vi "Blink_SDK_example.vi"() -> ()   [LabVIEW 2010]
uses:
  Blink_C_wrapper.dll
  ImageGen.dll
panel:
  out "ImgData 2":u8[](array[numeric])
  in  "Wait Timer":dbl=1000.0
  in  "Use External Triggers":bool
  out "BoardNum":i32
  out "ImgData":u8[](array[numeric])
  # "PCIe  LabVIEWSDK"
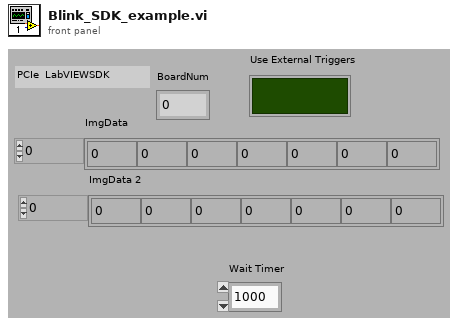
[diagram p1: front panel]
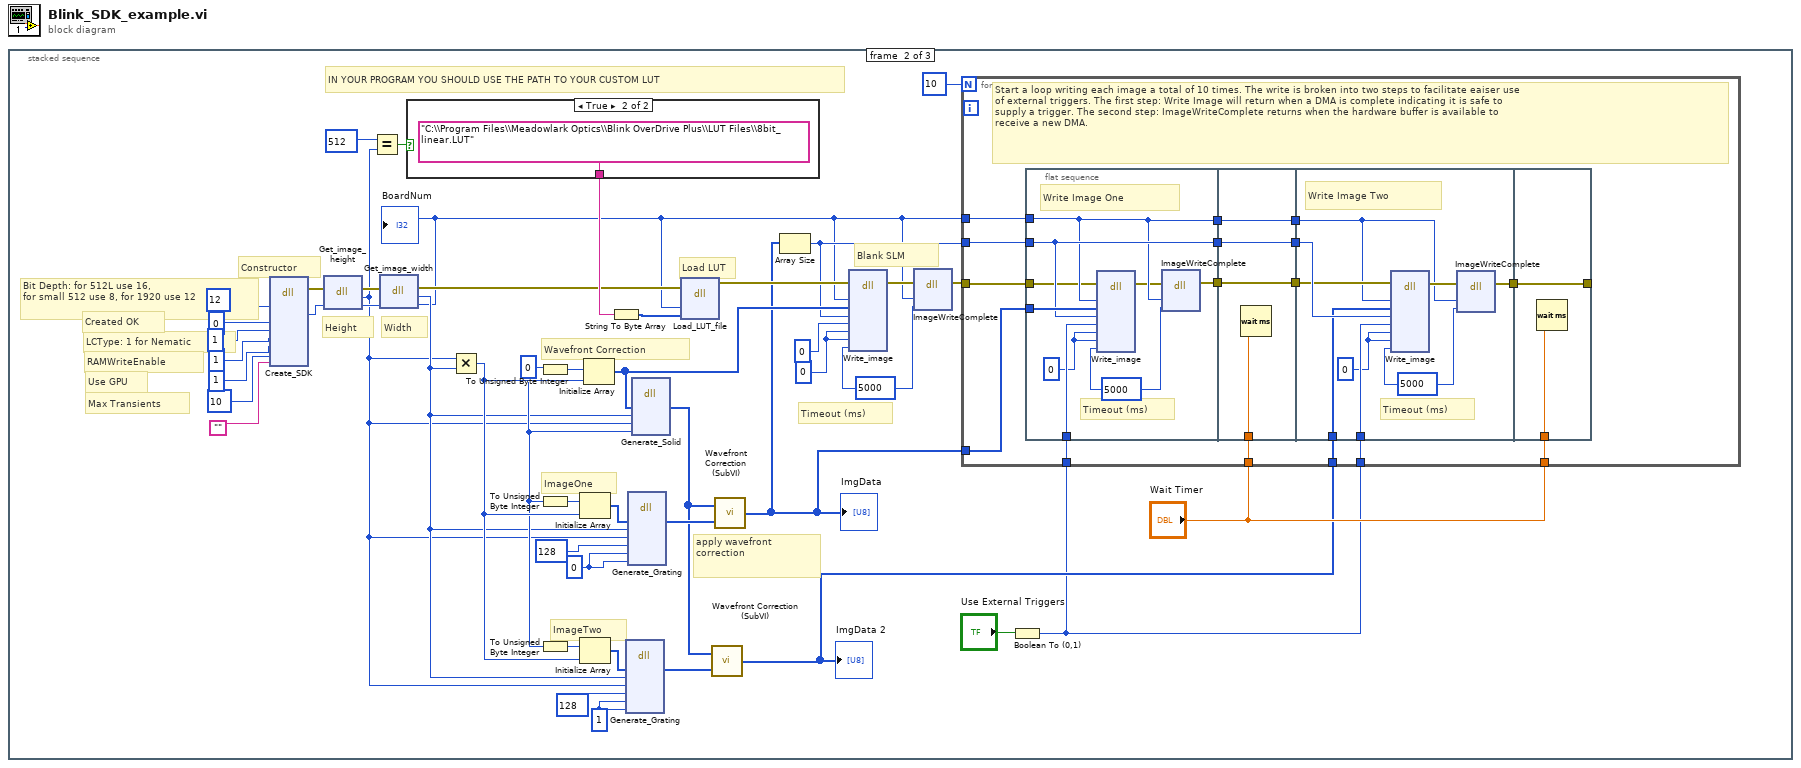
[diagram p0: block diagram]
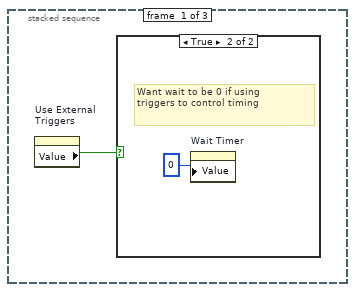
[diagram p2: hidden frame]
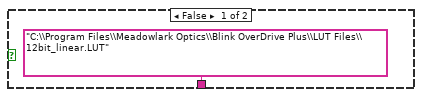
[diagram p4: hidden frame]
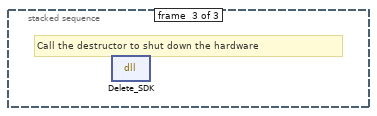
[diagram p5: hidden frame]
diagram:
  n1 = stacked-sequence {
    frame #0 {
      n2 = property on="Use External \nTriggers" class="Bool (strict)"() -> ("Value"=w1:bool)  [unwired: 2 in, 2 out]
      n3 = case shown="True" w1 {
        frame False {
        }
        frame True {
          # "Want wait to be 0 if using \ntriggers to control timing"
          n4 = property on="Wait Timer" class="DigNum (strict)"("Value"=0) -> ()  [unwired: 2 in, 2 out]
        }
      }
    }
    frame #1 {
      w14 = 5000
      w3 = 0
      w29 = 1
      w31 = 0
      w34 = 0
      # "Timeout (ms)"
      # "Blank SLM"
      # "IN YOUR PROGRAM YOU SHOULD USE THE PATH TO YOUR CUSTOM LUT"
      # "Load LUT"
      # "ImageTwo"
      # "ImageOne"
      # "Wavefront Correction"
      # "Width"
      # "Height"
      # "apply wavefront\ncorrection"
      # "Created OK"
      # "Max Transients"
      # "Use GPU"
      # "RAMWriteEnable"
      # "Bit Depth: for 512L use 16, \nfor small 512 use 8, for 1920 use 12"
      # "LCType: 1 for Nematic"
      # "Constructor"
      n5 = dll-call lib="C:/Meadowlark/Repos-git/MeadowlarkOverdrivePlus/src/Blink_SDK_example_grizzly/Blink_C_wrapper.dll" fn="Create_SDK"("SLM_bit_depth"=12, "constructed_ok"=0, "is_nematic_type"=1, "RAM_write_enable"=1, "use_GPU_if_available"=1, "max_transient_frames"=10, "static_regional_lut_file"="") -> (error out=w17:errorcluster, "n_boards_found"=w16:u64)  [unwired: 12 in, 1 out]
      n6 = dll-call lib="C:/Meadowlark/Repos-git/MeadowlarkOverdrivePlus/src/Blink_SDK_example_grizzly/Blink_C_wrapper.dll" fn="Get_image_height"(error in=w17, "Board"=w16) -> (error out=w39:errorcluster, "return type"=w20:i32, "Board"=w40:u32)  [unwired: 2 in, 1 out]
      n7 = Equal?(x=512, y=w20) -> (x = y?=w22:bool)
      n8 = dll-call lib="C:/Meadowlark/Repos-git/MeadowlarkOverdrivePlus/src/Blink_SDK_example_grizzly/Blink_C_wrapper.dll" fn="Get_image_width"(error in=w39, "Board"=w40) -> (error out=w12:errorcluster, "return type"=w27:i32, "Board"=w4:u32)  [unwired: 2 in, 1 out]
      "BoardNum" <- w4
      n9 = case shown="True" w22 {
        tunnel: ["C:\\Program Files\\Meadowlark Optics\\Blink OverDrive Plus\\LUT Files\\12bit_linear.LUT" "C:\\Program Files\\Meadowlark Optics\\Blink OverDrive Plus\\LUT Files\\8bit_linear.LUT"] -> w19
        frame False {
        }
        frame True {
        }
      }
      n10 = Multiply(x=w20, y=w27) -> (x*y=w38:i32)
      n11 = To Unsigned Byte Integer(number=w34) -> (unsigned 8bit integer=w37:u8)
      n12 = To Unsigned Byte Integer(number=w34) -> (unsigned 8bit integer=w36:u8)
      n13 = To Unsigned Byte Integer(number=w34) -> (unsigned 8bit integer=w35:u8)
      n14 = Initialize Array(w36, w38) -> (w33:u8[])
      n15 = Initialize Array(w35, w38) -> (w30:u8[])
      n16 = Initialize Array(w37, w38) -> (w9:u8[])
      n17 = String To Byte Array(string=w19) -> (unsigned byte array=w18:u8[])
      n18 = dll-call lib="C:/Meadowlark/Repos-git/MeadowlarkOverdrivePlus/src/Blink_SDK_example_grizzly/ImageGen.dll" fn="Generate_Grating"("Array"=w30, "Width"=w27, "Height"=w20, "Period"=128, "Increasing"=w29, "Horizontal"=w29) -> ("Array"=w24:u8[])  [unwired: 9 in, 2 out]
      n19 = dll-call lib="C:/Meadowlark/Repos-git/MeadowlarkOverdrivePlus/src/Blink_SDK_example_grizzly/ImageGen.dll" fn="Generate_Grating"("Array"=w33, "Width"=w27, "Height"=w20, "Period"=128, "Increasing"=w31, "Horizontal"=w31) -> ("Array"=w26:u8[])  [unwired: 9 in, 2 out]
      n20 = dll-call lib="C:/Meadowlark/Repos-git/MeadowlarkOverdrivePlus/src/Blink_SDK_example_grizzly/ImageGen.dll" fn="Generate_Solid"("Array"=w9, "Width"=w27, "Height"=w20, "PixelValue"=w34) -> ("Array"=w25:u8[])  [unwired: 7 in, 2 out]
      n21 = dll-call lib="C:/Meadowlark/Repos-git/MeadowlarkOverdrivePlus/src/Blink_SDK_example_grizzly/Blink_C_wrapper.dll" fn="Load_LUT_file"(error in=w12, "Board"=w4, "LUTPath"=w18) -> (error out=w11:errorcluster)  [unwired: 5 in, 1 out]
      n22 = call "Wavefront Correction (SubVI).vi"("Source Image Array"=w24, "Wavefront Correction"=w25) -> ("Corrected Image Array"=w23:u8[])
      "ImgData 2" <- w23
      n23 = call "Wavefront Correction (SubVI).vi"("Source Image Array"=w26, "Wavefront Correction"=w25) -> ("Corrected Image Array"=w8:u8[])
      "ImgData" <- w8
      n24 = Array Size(array=w8) -> (size(s)=w5:i32)
      n25 = dll-call lib="C:/Meadowlark/Repos-git/MeadowlarkOverdrivePlus/src/Blink_SDK_example_grizzly/Blink_C_wrapper.dll" fn="Write_image"(error in=w11, "board"=w4, "Image"=w9, "ImageSize"=w5, "WaitForTrigger"=0, "OutputPulseImageFlip"=w3, "OutputPulseImageRefresh"=w3, "timeout"=w14) -> (error out=w13:errorcluster)  [unwired: 10 in, 1 out]
      n26 = dll-call lib="C:/Meadowlark/Repos-git/MeadowlarkOverdrivePlus/src/Blink_SDK_example_grizzly/Blink_C_wrapper.dll" fn="ImageWriteComplete"(error in=w13, "board"=w4, "timeout"=w14) -> (error out=w10:errorcluster)  [unwired: 5 in, 1 out]
      n27 = Boolean To (0,1)(Boolean="Use External Triggers") -> (0, 1=w6:i16)
      n28 = for {
        N: 10 -> [_]
        tunnel: w4 -> [w67]
        tunnel: w5 -> [w66]
        tunnel: w23 -> [w65]
        tunnel: "Wait Timer" -> [w60]
        tunnel: "Wait Timer" -> [w59]
        tunnel: w10 -> [w55]
        tunnel: w8 -> [w54]
        tunnel: w6 -> [w53]
        tunnel: w6 -> [w52]
        # "Start a loop writing each image a total of 10 times. The write is broken into two steps to facilitate eaiser use\nof external triggers. The first step: Write Image will return when a DMA is complete indicating it is safe to \nsupply a trigger. The second step: ImageWriteComplete returns when the hardware buffer is available to \nreceive a new DMA."
        n29 = flat-sequence {
          tunnel: w67 -> [w74]
          tunnel: w54 -> [w76]
          tunnel: w66 -> [w75]
          tunnel: [w74] -> w64
          tunnel: [w75] -> w62
          tunnel: [w71] -> w57
          tunnel: w55 -> [w70]
          tunnel: w53 -> [w69]
          tunnel: w64 -> [w80]
          tunnel: [w80] -> w63
          tunnel: w62 -> [w79]
          tunnel: [w79] -> w61
          tunnel: w60 -> [w78]
          tunnel: [w77] -> w58
          tunnel: w57 -> [w77]
          tunnel: w63 -> [w84]
          tunnel: w61 -> [w89]
          tunnel: w65 -> [w88]
          tunnel: w58 -> [w87]
          tunnel: [w85] -> w56
          tunnel: w52 -> [w82]
          tunnel: w59 -> [w91]
          tunnel: [w90] -> _
          tunnel: w56 -> [w90]
          frame #0 {
            w73 = 5000
            w68 = 0
            # "Timeout (ms)"
            # "Write Image One"
            n30 = dll-call lib="C:/Meadowlark/Repos-git/MeadowlarkOverdrivePlus/src/Blink_SDK_example_grizzly/Blink_C_wrapper.dll" fn="Write_image"(error in=w70, "board"=w74, "Image"=w76, "ImageSize"=w75, "WaitForTrigger"=w69, "OutputPulseImageFlip"=w68, "OutputPulseImageRefresh"=w68, "timeout"=w73) -> (error out=w72:errorcluster)  [unwired: 10 in, 1 out]
            n31 = dll-call lib="C:/Meadowlark/Repos-git/MeadowlarkOverdrivePlus/src/Blink_SDK_example_grizzly/Blink_C_wrapper.dll" fn="ImageWriteComplete"(error in=w72, "board"=w74, "timeout"=w73) -> (error out=w71:errorcluster)  [unwired: 5 in, 1 out]
          }
          frame #1 {
            n32 = Wait (ms)(milliseconds to wait=w78) -> ()  [unwired: 1 out]
          }
          frame #2 {
            w83 = 5000
            w81 = 0
            # "Timeout (ms)"
            # "Write Image Two"
            n33 = dll-call lib="C:/Meadowlark/Repos-git/MeadowlarkOverdrivePlus/src/Blink_SDK_example_grizzly/Blink_C_wrapper.dll" fn="Write_image"(error in=w87, "board"=w84, "Image"=w88, "ImageSize"=w89, "WaitForTrigger"=w82, "OutputPulseImageFlip"=w81, "OutputPulseImageRefresh"=w81, "timeout"=w83) -> (error out=w86:errorcluster)  [unwired: 10 in, 1 out]
            n34 = dll-call lib="C:/Meadowlark/Repos-git/MeadowlarkOverdrivePlus/src/Blink_SDK_example_grizzly/Blink_C_wrapper.dll" fn="ImageWriteComplete"(error in=w86, "board"=w84, "timeout"=w83) -> (error out=w85:errorcluster)  [unwired: 5 in, 1 out]
          }
          frame #3 {
            n35 = Wait (ms)(milliseconds to wait=w91) -> ()  [unwired: 1 out]
          }
        }
      }
    }
    frame #2 {
      # "Call the destructor to shut down the hardware"
      n36 = dll-call lib="C:/Meadowlark/Repos-git/MeadowlarkOverdrivePlus/src/Blink_SDK_example_grizzly/Blink_C_wrapper.dll" fn="Delete_SDK"() -> ()  [unwired: 4 in, 2 out]
    }
  }
